vi "Reset Write Statistics.vi"(8 "error in (no error)":errorcluster, 11 "Main in":refnum<class "Main.lvclass">) -> (0 "error out":errorcluster, 3 "Main out":refnum<class "Main.lvclass">)   [LabVIEW 2025, in "Main.lvlib" / "Main.lvclass"]
uses:
  Main.lvclass
  Main.lvclass/Main.ctl
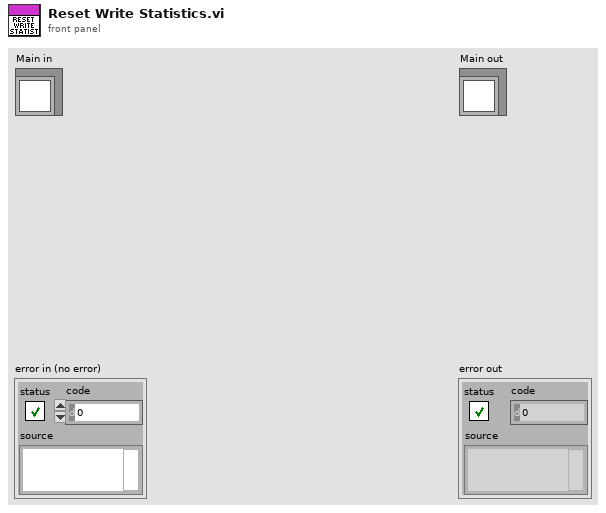
[diagram p1: front panel]
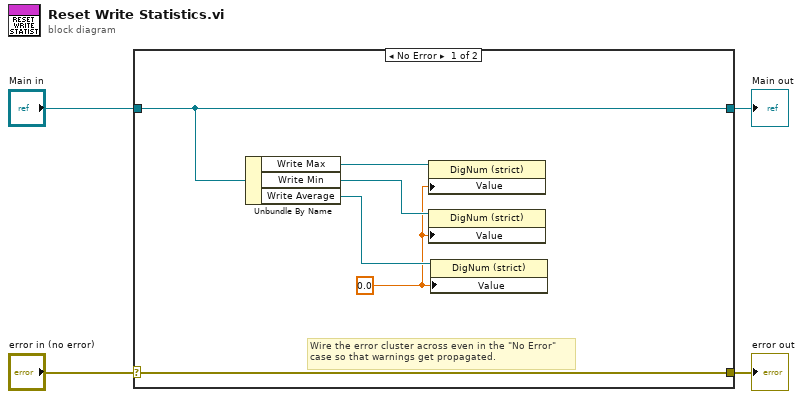
[diagram p0: block diagram]
diagram:
  n1 = case shown="No Error" "error in (no error)" {
    selector: "error in (no error)" -> [w10 w12]
    tunnel: [w10 w12] -> w3
    tunnel: [w5 w11] -> w1
    tunnel: "Main in" -> [w5 w11]
    frame No Error {
      w6 = 0.0 ("Value")
      # "Wire the error cluster across even in the \"No Error\"\ncase so that warnings get propagated."
      n2 = Unbundle By Name(w5) -> ("Write Max"=w9:refnum<vi>, "Write Min"=w8:refnum<vi>, "Write Average"=w7:refnum<vi>)
      n3 = property class="DigNum (strict)"(reference=w9, "Value"=w6) -> ()  [unwired: 1 in, 2 out]
      n4 = property class="DigNum (strict)"(reference=w8, "Value"=w6) -> ()  [unwired: 1 in, 2 out]
      n5 = property class="DigNum (strict)"(reference=w7, "Value"=w6) -> ()  [unwired: 1 in, 2 out]
    }
    frame Error {
    }
  }
  "error out" <- w3
  "Main out" <- w1
